vi "ModuloTeste.vi"(0 "IA State Input":T2, 1 "atacando ao contrário?":bool=TRUE, 2 "Dribble":bool, 3 "angulo":dbl=90.0 format="%#_13g", 4 "GoTo point":dbl[](array[numeric])=[0.0, 0.0, 0.0], 5 "points 3":cluster{"x":dbl, "y":dbl}[](array[cluster])=[{"x"=0.0, "y"=0.0}, {"x"=1000.0, "y"=1000.0}, {"x"=-1000.0, "y"=1000.0}], 6 "Kick?":bool, 7 "Kicker":T1="None", 8 "speed print selector":u32, 9 "ZigZag 0":T1="None", 11 "gravando":bool=TRUE, 12 "Vel_kick":dbl=5.0 format="%#_13g", 13 "Goto":T1="None", 18 "output xy":dbl=2.0, 19 "output angle":dbl=2.0) -> (14 "IA State Output":T2, 15 "ball":dbl(graph), 17 "Robot":dbl(graph))   [LabVIEW 2017]
uses:
  Core/AI Input.ctl
  Core/AI Robot.ctl
  Functions Enum.ctl
  AttackerStates.ctl
  Core/AI Ball.ctl
  Core/Field Size.ctl
  Core/AI Judge.ctl
  Command Enum.ctl
  Util/Events/Events.ctl
  Util/Select None or Robot.ctl
  <vilib>/Analysis/_algsub.llb/Real Vector Norm.vi
  <vilib>/Analysis/NI_AALPro.lvlib
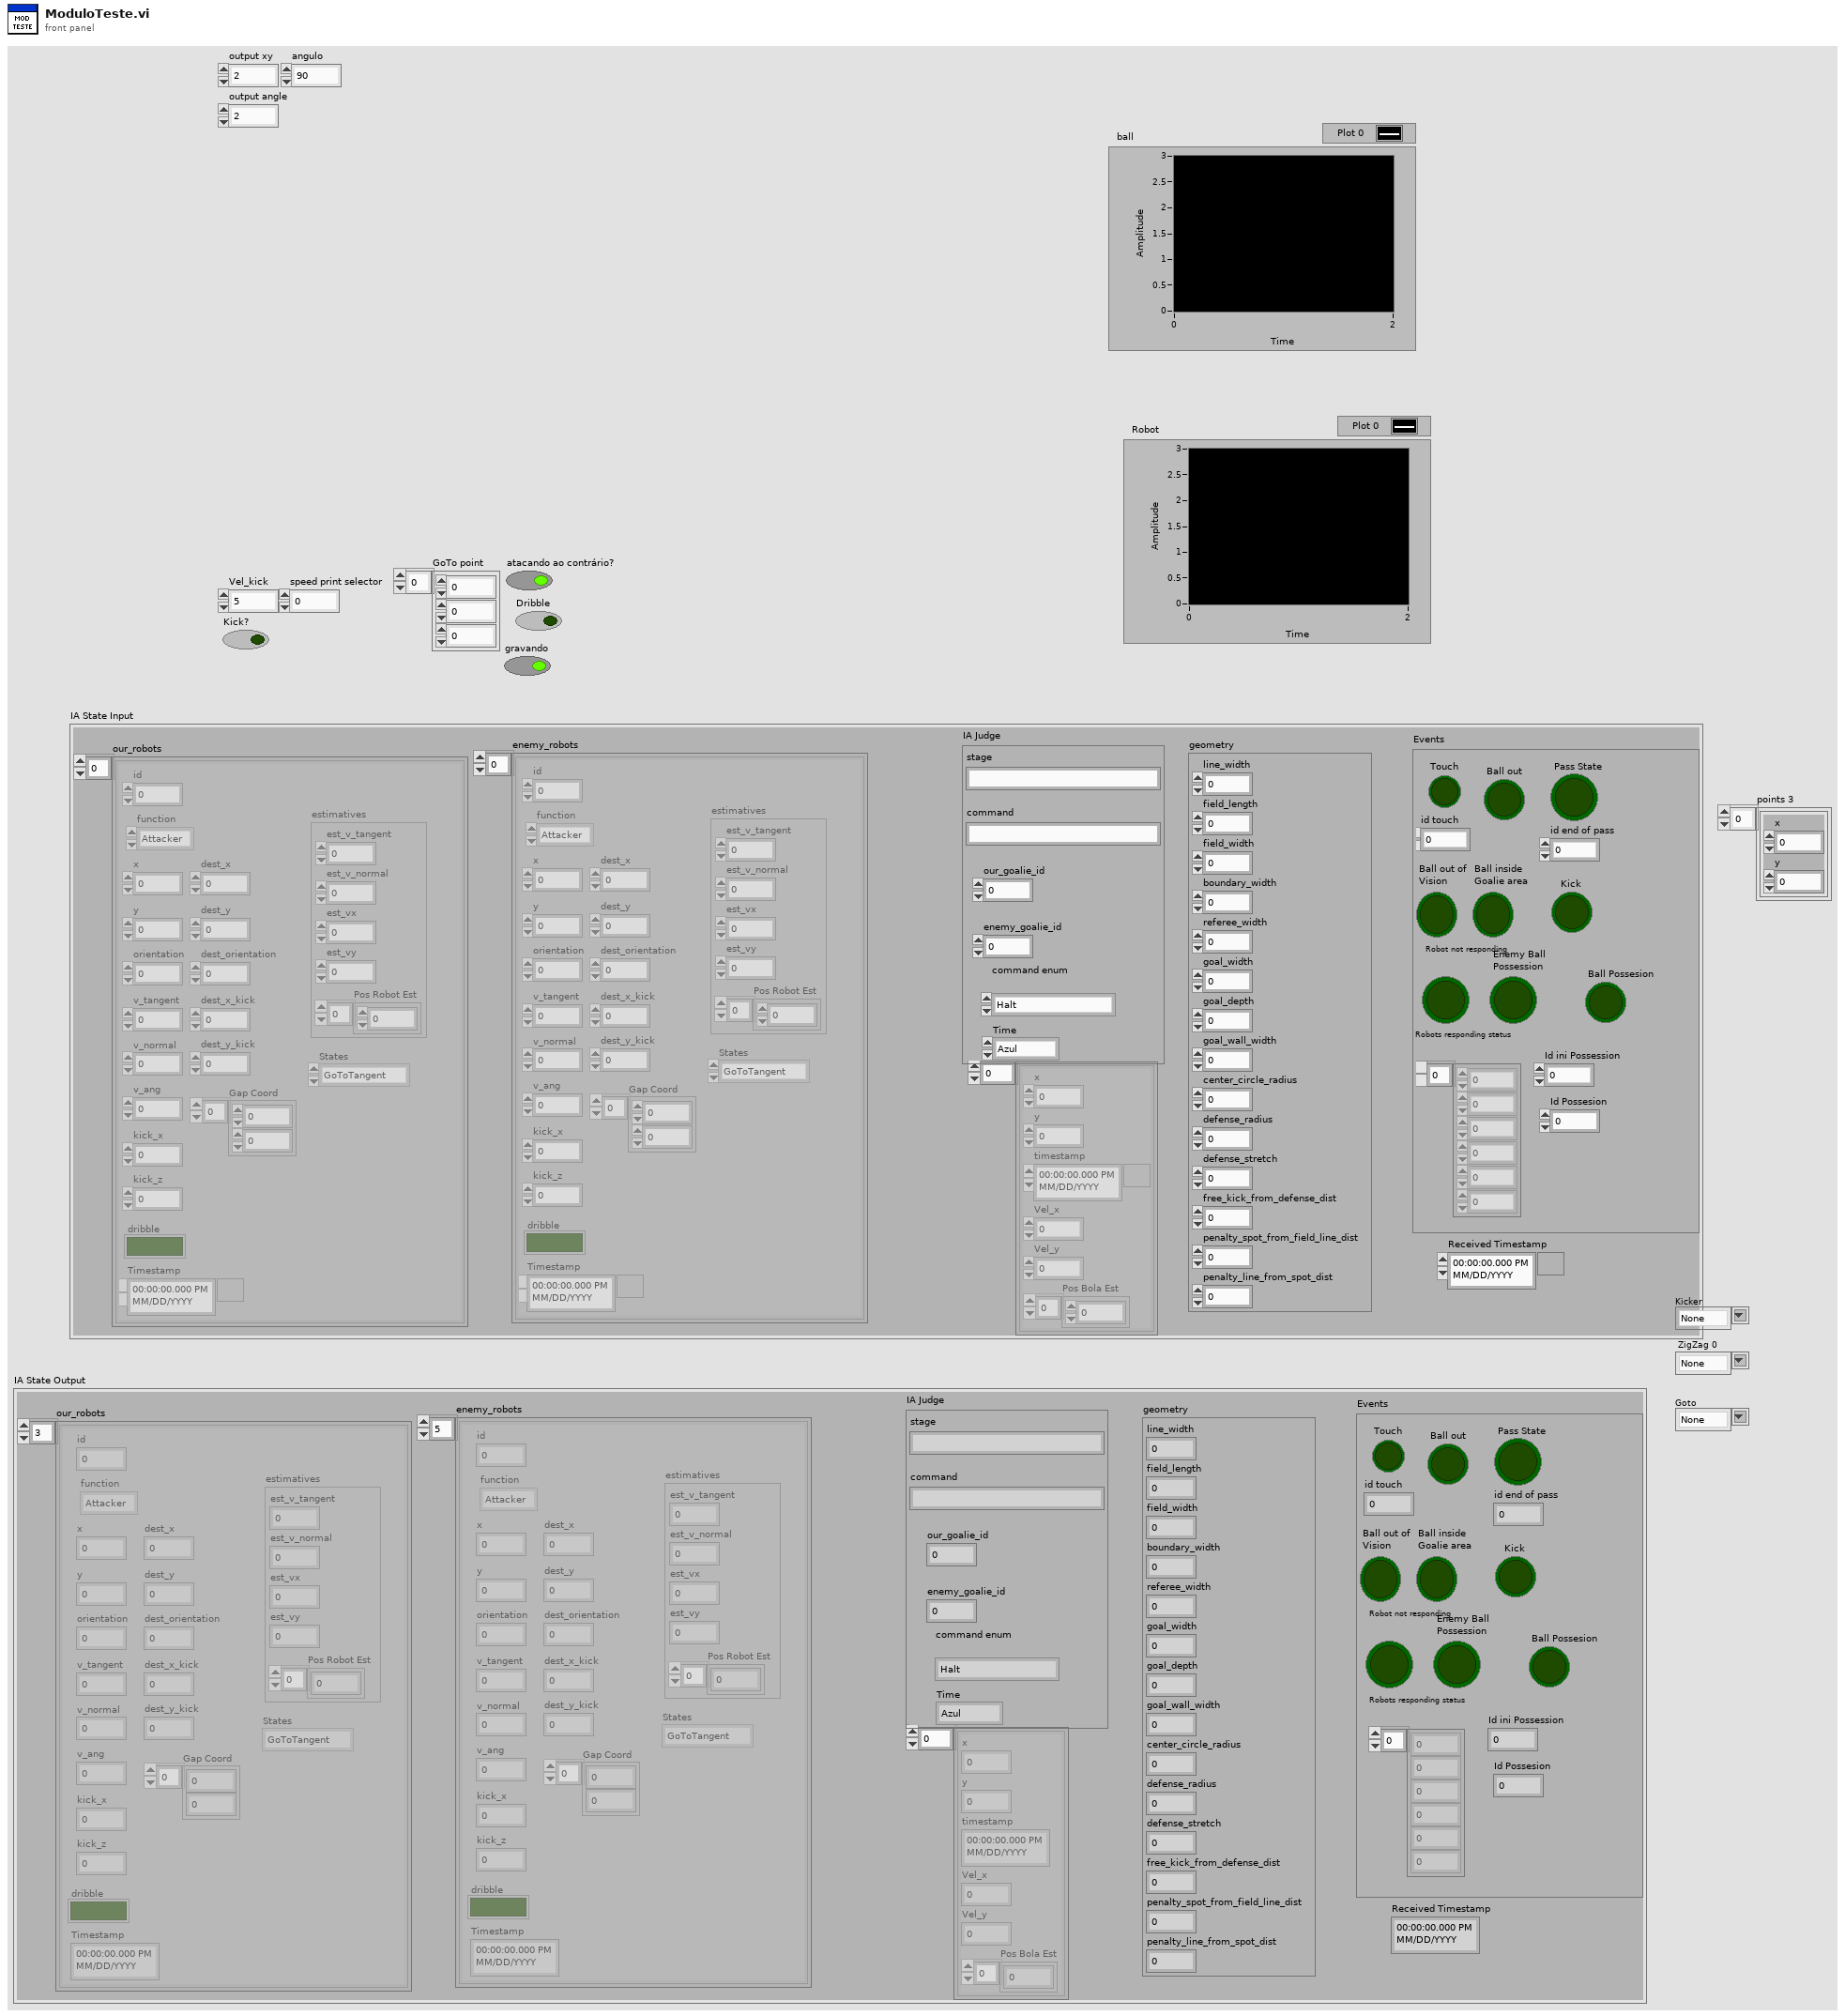
[diagram p1: front panel]
types:
  T1 = typedef "Select None or Robot.ctl" = string
  T2 = typedef "AI Input.ctl" = cluster{"our_robots":T3[], "enemy_robots":T3[], "balls":T6[], "geometry":T7, "IA Judge":T8, "Received Timestamp":timestamp, "Events":T10}
  T3 = typedef "AI Robot.ctl" = cluster{"id":u32, "function":T4, "x":dbl, "y":dbl, "orientation":dbl, "v_tangent":dbl, "v_normal":dbl, "v_ang":dbl, "kick_x":dbl, "kick_z":dbl, "dribble":bool, "Timestamp":timestamp, "dest_x":dbl, "dest_y":dbl, "dest_orientation":dbl, "estimatives":cluster{"est_v_tangent":dbl, "est_v_normal":dbl, "est_vx":dbl, "est_vy":dbl, "Pos Robot Est":dbl[]}, "dest_x_kick":dbl, "dest_y_kick":dbl, "Gap Coord":dbl[], "States":T5}
  T4 = typedef "Functions Enum.ctl" = enum16{"Attacker", "Goalie", "Defender", "Striker", "Goto 0", "Dummy", "Kicker", "ZigZag"}
  T5 = typedef "AttackerStates.ctl" = enum16{"Pass", "GoToTangent", "BallGetting", "GoToKick", ""}
  T6 = typedef "AI Ball.ctl" = cluster{"x":dbl, "y":dbl, "timestamp":timestamp, "Vel_x":dbl, "Vel_y":dbl, "Pos Bola Est":dbl[]}
  T7 = typedef "Field Size.ctl" = cluster{"line_width":u32, "field_length":u32, "field_width":u32, "boundary_width":u32, "referee_width":u32, "goal_width":u32, "goal_depth":u32, "goal_wall_width":u32, "center_circle_radius":u32, "defense_radius":u32, "defense_stretch":u32, "free_kick_from_defense_dist":u32, "penalty_spot_from_field_line_dist":u32, "penalty_line_from_spot_dist":u32}
  T8 = typedef "AI Judge.ctl" = cluster{"stage":string, "command":string, "our_goalie_id":dbl, "enemy_goalie_id":dbl, "command enum":T9, "Time":enum16{"Azul", "Amarelo"}}
  T9 = typedef "Command Enum.ctl" = enum16{"Halt", "Stop", "Force Start", "PKA Normal Start", "Prepare Kickoff Ally", "PKE Normal Start", "Prepare Kickoff Enemy", "Prepare Penalty Ally", "PPA Normal Start", "Prepare Penalty Enemy", "PPE Normal Start", "Direct Free Enemy", "Direct Free Ally", "Indirect Free Enemy", "Indirect Free Ally", "Timeout Enemy", "Timeout Ally", "Goal Enemy", "Goal Ally", "Ball Placement Enemy", "Ball Placement Ally", "Normal Half Time", "Extra Time Break", "Extra Half Time", "None", "Post Game"}
  T10 = typedef "Events.ctl" = cluster{"Touch":bool, "Ball out":bool, "id touch":dbl, "Ball out of \nVision":bool, "Ball inside \nGoalie area":bool, "Robot not responding":bool, "Robots responding status":dbl[], "Enemy Ball \nPossession":bool, "Pass State":bool, "id end of pass":dbl, "Kick":bool, "Id ini Possession":dbl, "Ball Possesion":bool, "Id Possesion":dbl}
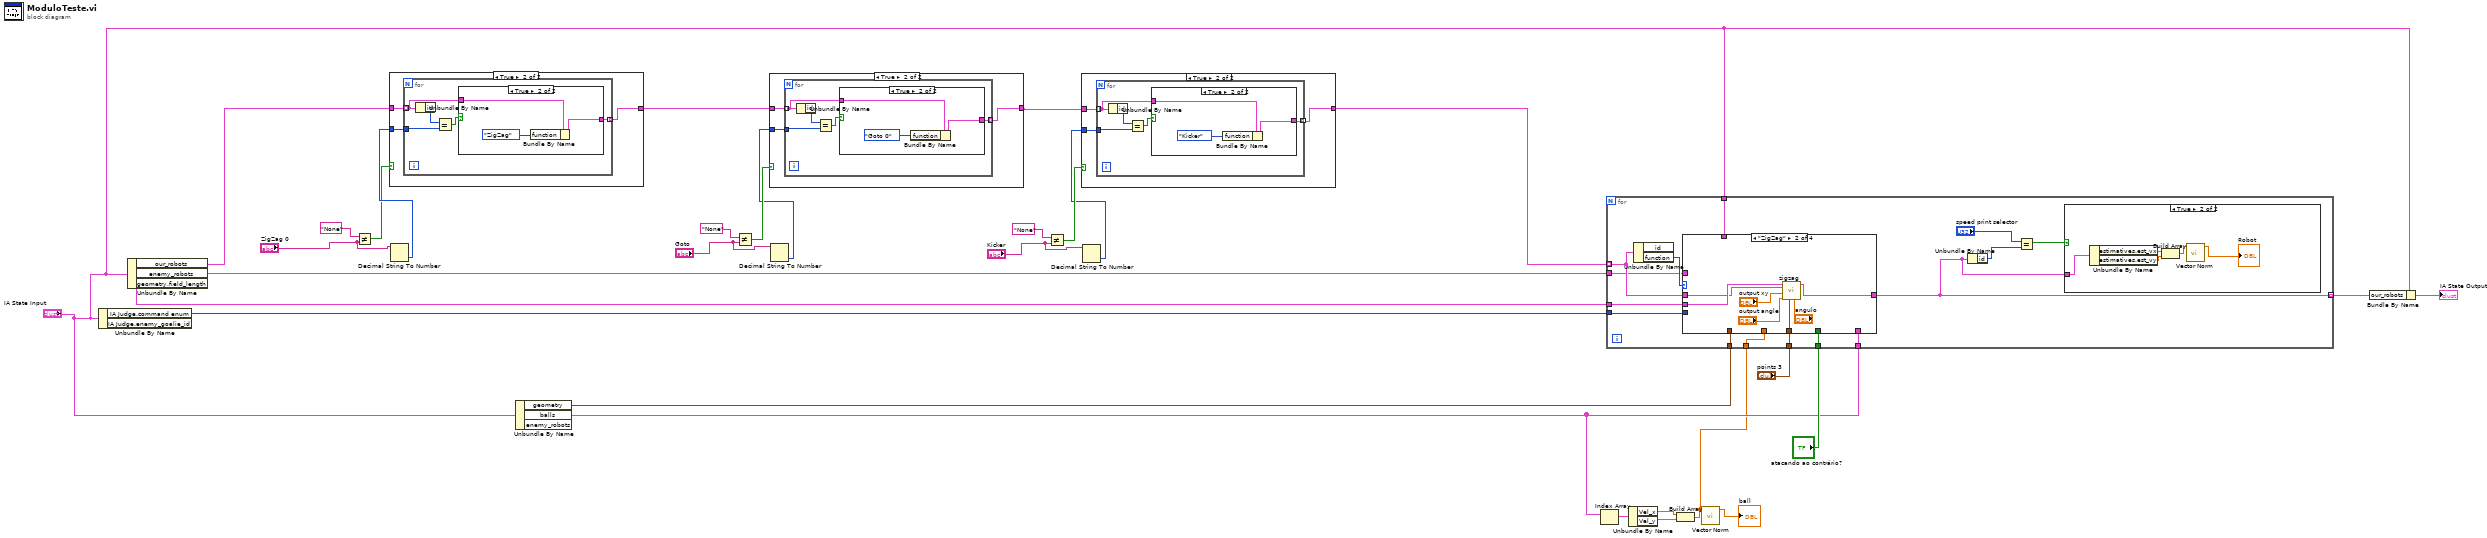
[diagram p0: block diagram]
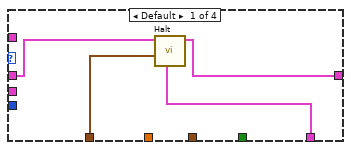
[diagram p9: hidden frame]
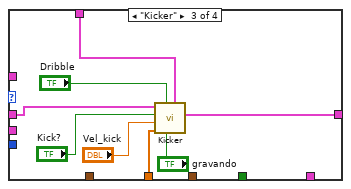
[diagram p10: hidden frame]
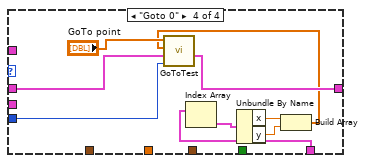
[diagram p11: hidden frame]
diagram:
  n1 = Unbundle By Name("IA State Input") -> ("IA Judge.command enum"=w30:T9)  [unwired: 1 out]
  n2 = Unbundle By Name("IA State Input") -> ("our_robots"=w21:T3[], "enemy_robots"=w26:T3[])  [unwired: 1 out]
  n3 = Not Equal?(x="None", y="ZigZag 0") -> (x != y?=w23:bool)
  n4 = Decimal String To Number(string="ZigZag 0") -> (number=w24:i32)  [unwired: 2 in, 1 out]
  n5 = case shown="True" w23 {
    tunnel: w24 -> [_ w34]
    tunnel: [w31 w33] -> w18
    tunnel: w21 -> [w31 w32]
    frame False {
    }
    frame True {
      n6 = for {
        tunnel: w34 -> [w38]
        tunnel: [w36] -> w33 mode=indexing
        tunnel: w32 -> [w35] mode=indexing
        n7 = Unbundle By Name(w35) -> ("id"=w39:u32)
        n8 = Equal?(x=w39, y=w38) -> (x = y?=w37:bool)
        n9 = case shown="True" w37 {
          tunnel: [w40 w43] -> w36
          tunnel: w35 -> [w40 w41]
          frame False {
          }
          frame True {
            n10 = Bundle By Name(cluster=w41, "function"=Functions_Enum."ZigZag") -> (w43:T3)
          }
        }
      }
    }
  }
  n11 = Unbundle By Name("IA State Input") -> ("geometry"=w27:T7, "balls"=w8:T6[])  [unwired: 1 out]
  n12 = Not Equal?(x="None", y="Goto") -> (x != y?=w20:bool)
  n13 = Decimal String To Number(string="Goto") -> (number=w15:i32)  [unwired: 2 in, 1 out]
  n14 = case shown="True" w20 {
    tunnel: w15 -> [_ w47]
    tunnel: [w44 w46] -> w10
    tunnel: w18 -> [w44 w45]
    frame False {
    }
    frame True {
      n15 = for {
        tunnel: w47 -> [w51]
        tunnel: [w49] -> w46 mode=indexing
        tunnel: w45 -> [w48] mode=indexing
        n16 = Unbundle By Name(w48) -> ("id"=w52:u32)
        n17 = Equal?(x=w52, y=w51) -> (x = y?=w50:bool)
        n18 = case shown="True" w50 {
          tunnel: [w53 w56] -> w49
          tunnel: w48 -> [w53 w54]
          frame False {
          }
          frame True {
            n19 = Bundle By Name(cluster=w54, "function"=Functions_Enum."Goto 0") -> (w56:T3)
          }
        }
      }
    }
  }
  n20 = Not Equal?(x="None", y="Kicker") -> (x != y?=w14:bool)
  n21 = Decimal String To Number(string="Kicker") -> (number=w11:i32)  [unwired: 2 in, 1 out]
  n22 = case shown="True" w14 {
    tunnel: w11 -> [_ w60]
    tunnel: [w57 w59] -> w9
    tunnel: w10 -> [w57 w58]
    frame False {
    }
    frame True {
      n23 = for {
        tunnel: w60 -> [w64]
        tunnel: [w62] -> w59 mode=indexing
        tunnel: w58 -> [w61] mode=indexing
        n24 = Unbundle By Name(w61) -> ("id"=w65:u32)
        n25 = Equal?(x=w65, y=w64) -> (x = y?=w63:bool)
        n26 = case shown="True" w63 {
          tunnel: [w66 w69] -> w62
          tunnel: w61 -> [w66 w67]
          frame False {
          }
          frame True {
            n27 = Bundle By Name(cluster=w67, "function"=Functions_Enum."Kicker") -> (w69:T3)
          }
        }
      }
    }
  }
  n28 = Index Array(array=w8) -> (element=w7:T6)  [unwired: 1 in]
  n29 = Unbundle By Name(w7) -> ("Vel_x"=w6:dbl, "Vel_y"=w5:dbl)
  n30 = Build Array(w6, w5) -> (w2:dbl[])
  n31 = for {
    tunnel: w9 -> [w83] mode=indexing
    tunnel: [w73] -> w29 mode=indexing
    tunnel: w30 -> [w82]
    tunnel: "IA State Input" -> [w81]
    tunnel: w27 -> [w80]
    tunnel: w8 -> [w79]
    tunnel: w26 -> [w78]
    tunnel: "atacando ao contrário?" -> [w77]
    tunnel: "points 3" -> [w72]
    tunnel: w2 -> [w71]
    tunnel: "IA State Input" -> [w70]
    n32 = Unbundle By Name(w83) -> ("function"=w84:T4)  [unwired: 1 out]
    n33 = case shown="\"ZigZag\"" w84 {
      tunnel: w83 -> [w93 w98 w107 w116]
      tunnel: [w92 w100 w108 w115] -> w73
      tunnel: w82 -> [_ _ _ w114]
      tunnel: w81 -> [_ w99 _ _]
      tunnel: w80 -> [w91 _ _ _]
      tunnel: w79 -> [w90 _ _ w113]
      tunnel: w78 -> [_ _ _ _]
      tunnel: w77 -> [_ _ _ _]
      tunnel: w72 -> [_ w97 _ _]
      tunnel: w71 -> [_ _ w103 _]
      tunnel: w70 -> [_ _ w102 _]
      frame Default {
        n34 = call "Halt.vi"("balls"=w90, "Field Size in"=w91, "Robot in"=w93) -> ("Robot out"=w92:T3)  [unwired: 8 in]
      }
      frame "ZigZag" {
        n35 = call "zigzag.vi"("angulo"="angulo", "points 3"=w97, "output angle"="output angle", "output xy"="output xy", "Current Robot"=w98, "Al Input"=w99) -> ("Output Robot"=w100:T3)  [unwired: 5 in]
      }
      frame "Kicker" {
        n36 = call "Kicker.vi"("IA State Input"=w102, "gravar"="gravando", "Dribble"="Dribble", "Ball velocity"=w103, "Vel_kick"="Vel_kick", "Kick?"="Kick?", "Robot in"=w107) -> ("output cluster"=w108:T3)  [unwired: 4 in]
      }
      frame "Goto 0" {
        n37 = Index Array(array=w113) -> (element=w112:T6)  [unwired: 1 in]
        n38 = Unbundle By Name(w112) -> ("x"=w111:dbl, "y"=w110:dbl)
        n39 = Build Array(w111, w110) -> (w109:dbl[])
        n40 = call "GoToTest.vi"("command\nenum"=w114, "Robot In"=w116, "Ball"=w109, "GoTo point"="GoTo point") -> ("Robot Out"=w115:T3)  [unwired: 7 in]
      }
    }
    n41 = Unbundle By Name(w73) -> ("id"=w76:u32)
    n42 = Equal?(x="speed print selector", y=w76) -> (x = y?=w74:bool)
    n43 = case shown="True" w74 {
      tunnel: w73 -> [_ w89]
      frame False {
      }
      frame True {
        n44 = Unbundle By Name(w89) -> ("estimatives.est_vx"=w88:dbl, "estimatives.est_vy"=w87:dbl)
        n45 = Build Array(w88, w87) -> (w86:dbl[])
        n46 = call-poly <vilib>:"Vector Norm.vi"("Input Vector"=w86) -> ("norm"=→"Robot":dbl)  [unwired: 9 in, 1 out]
      }
    }
  }
  n47 = call-poly <vilib>:"Vector Norm.vi"("Input Vector"=w2) -> ("norm"=→"ball":dbl)  [unwired: 9 in, 1 out]
  n48 = Bundle By Name(cluster="IA State Input", "our_robots"=w29) -> (→"IA State Output":T2)
